vi "Function1.vi"   [LabVIEW 2016, in "Test.lvrbt"]
uses:
  Test.lvrbt
  <vilib>/NXT/Block Support/NXT_InputPort.ctl
  <vilib>/NXT/Hardware/Plugins/Tetrix DC Motor/TetrixDCMotorAddress.ctl
  <vilib>/NXT/Hardware/Plugins/Tetrix 180 deg Servo/Tetrix180ServoAddress.ctl
  <vilib>/NXT/NXTIO Xnodes/NXTIONodeSubVIs/TETRIX IO Move Servos.vi
  <vilib>/NXT/Dual Mode Library/Waits/Wait_Num.vi
  <vilib>/NXT/NXTIO Xnodes/NXTIONodeSubVIs/TETRIX IO Move DC Motors.vi
  <vilib>/NXT/NXTIO Xnodes/NXTIONodeSubVIs/TETRIX IO Stop DC Motors.vi
  <vilib>/NXT/Dual Mode Library/Waits/Wait_EV3_Ultrasonic_Centimeter_Closer.vi
  <vilib>/NXT/Dual Mode Library/Waits/Wait_Touch.vi
  <vilib>/NXT/Dual Mode Library/Waits/Wait_LetGo.vi
  <vilib>/NXT/NXTIO Xnodes/AddressXNode/NXTIOAddress.xnode
  <vilib>/NXT/Subs/LVHSConnector.ctl
  <vilib>/NXT/NXTIO Xnodes/NXTIOXNode/NXTIO.xnode
  <vilib>/NXT/LegoClasses/BrickReference/BrickReference.lvclass
types:
  T1 = typedef "NXT_InputPort.ctl" = u32
  T2 = typedef "Tetrix180ServoAddress.ctl" = i32
  T3 = cluster{"Tetrix180Servo":T2, "Tetrix180Servo":T2, "Tetrix180Servo":T2, "Tetrix180Servo":T2, "Tetrix180Servo":T2}
  T4 = typedef "LVHSConnector.ctl" = refnum<class "BrickReference.lvclass">
  T5 = typedef "TetrixDCMotorAddress.ctl" = i32
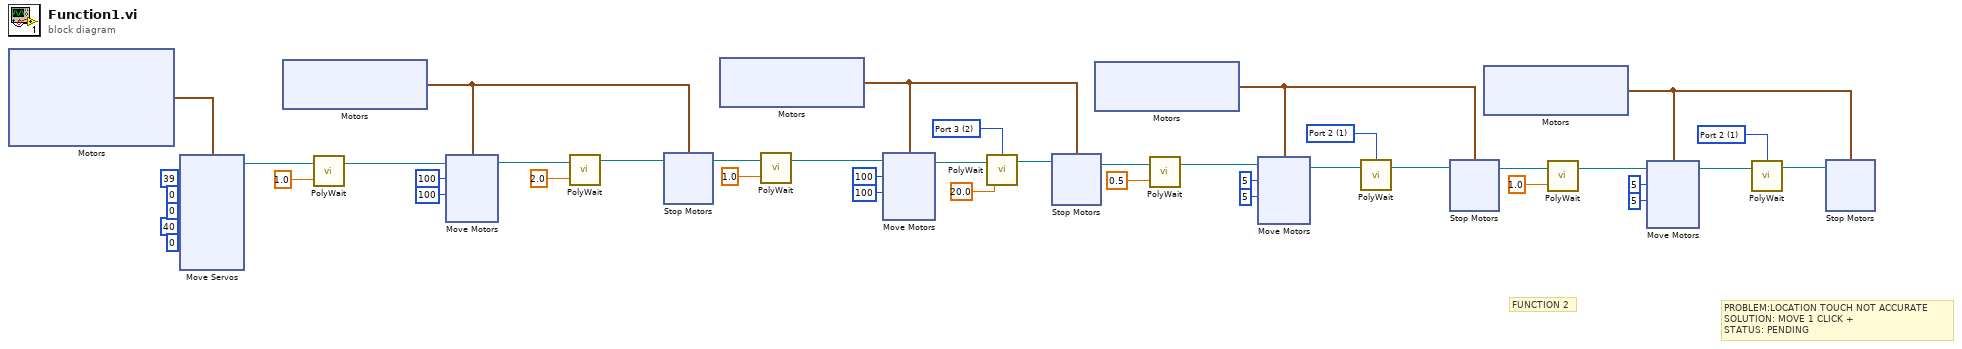
[diagram p0: block diagram]
diagram:
  w12 = T1 1 items=["Port 1", "Port 2", "Port 3", "Port 4"] ("Port (Port 1)")
  w21 = T1 1 items=["Port 1", "Port 2", "Port 3", "Port 4"] ("Port (Port 1)")
  w30 = T1 2 items=["Port 1", "Port 2", "Port 3", "Port 4"] ("Port (Port 1)")
  # "PROBLEM:LOCATION TOUCH NOT ACCURATE\nSOLUTION: MOVE 1 CLICK +\nSTATUS: PENDING"
  # "FUNCTION 2"
  n1 = xnode "Motors"() -> ("Motor"=w9:T3)
  n2 = xnode "Move Servos"("Position 5"=u8 0, "Position 4"=u8 40, "Position 3"=u8 0, "Position 2"=u8 0, "Position 1"=u8 39, "Motors"=w9) -> ("NXT/EV3"=w2:T4)  [unwired: 1 in]
  n3 = xnode "Motors"() -> ("Motor"=w38:cluster{"TetrixDCMotor":T5, "TetrixDCMotor":T5})
  n4 = call-poly <vilib>:"PolyWait.vi"("Time (1 sec)"=sgl 1.0, "NXT/EV3"=w2) -> ("NXT/EV3"=w1:T4)  [unwired: 2 in]
  n5 = xnode "Move Motors"("Power/Speed 1"=i8 100, "Motors"=w38, "NXT/EV3"=w1, "Power/Speed 2"=i8 100) -> ("NXT/EV3"=w43:T4)
  n6 = call-poly <vilib>:"PolyWait.vi"("Time (1 sec)"=sgl 2.0, "NXT/EV3"=w43) -> ("NXT/EV3"=w39:T4)  [unwired: 2 in]
  n7 = xnode "Stop Motors"("Motors"=w38, "NXT/EV3"=w39) -> ("NXT/EV3"=w36:T4)
  n8 = xnode "Motors"() -> ("Motor"=w28:cluster{"TetrixDCMotor":T5, "TetrixDCMotor":T5})
  n9 = call-poly <vilib>:"PolyWait.vi"("Time (1 sec)"=sgl 1.0, "NXT/EV3"=w36) -> ("NXT/EV3"=w33:T4)  [unwired: 2 in]
  n10 = xnode "Move Motors"("Power/Speed 2"=i8 100, "Power/Speed 1"=i8 100, "Motors"=w28, "NXT/EV3"=w33) -> ("NXT/EV3"=w32:T4)
  n11 = call-poly <vilib>:"PolyWait.vi"("Centimeters (40)"=sgl 20.0, "NXT/EV3"=w32, "Port (Port 1)"=w30) -> ("NXT/EV3"=w29:T4)  [unwired: 1 in]
  n12 = xnode "Stop Motors"("Motors"=w28, "NXT/EV3"=w29) -> ("NXT/EV3"=w24:T4)
  n13 = xnode "Motors"() -> ("Motor"=w19:cluster{"TetrixDCMotor":T5, "TetrixDCMotor":T5})
  n14 = call-poly <vilib>:"PolyWait.vi"("Time (1 sec)"=sgl 0.5, "NXT/EV3"=w24) -> ("NXT/EV3"=w23:T4)  [unwired: 2 in]
  n15 = xnode "Move Motors"("Power/Speed 2"=i8 5, "Power/Speed 1"=i8 5, "Motors"=w19, "NXT/EV3"=w23) -> ("NXT/EV3"=w22:T4)
  n16 = call-poly <vilib>:"PolyWait.vi"("NXT/EV3"=w22, "Port (Port 1)"=w21) -> ("NXT/EV3"=w20:T4)  [unwired: 2 in]
  n17 = xnode "Stop Motors"("Motors"=w19, "NXT/EV3"=w20) -> ("NXT/EV3"=w15:T4)
  n18 = xnode "Motors"() -> ("Motor"=w10:cluster{"TetrixDCMotor":T5, "TetrixDCMotor":T5})
  n19 = call-poly <vilib>:"PolyWait.vi"("Time (1 sec)"=sgl 1.0, "NXT/EV3"=w15) -> ("NXT/EV3"=w14:T4)  [unwired: 2 in]
  n20 = xnode "Move Motors"("Power/Speed 2"=i8 5, "Power/Speed 1"=i8 5, "Motors"=w10, "NXT/EV3"=w14) -> ("NXT/EV3"=w13:T4)
  n21 = call-poly <vilib>:"PolyWait.vi"("NXT/EV3"=w13, "Port (Port 1)"=w12) -> ("NXTEV3"=w11:T4)  [unwired: 2 in]
  n22 = xnode "Stop Motors"("Motors"=w10, "NXT/EV3"=w11) -> ()  [unwired: 1 out]
